vi "Set_DoublePulse_Delay.vi"(8 "error in":errorcluster, 9 "WaitForReady":bool, 10 "InputParams.":variant) -> (0 "error out":errorcluster, 2 "DP_StagePos.":variant)   [LabVIEW 2013]
uses:
  <instrlib>/ESP300/Public/Data/ESP300_State.ctl
  <instrlib>/ESP300/ESP300.lvlib
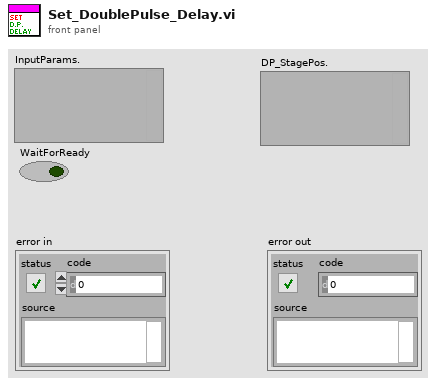
[diagram p1: front panel]
types:
  T1 = cluster{"MotionStageRefs":refnum<queue>, "Axis#":i32, "Delay(ps)":dbl, "ZeroDelay_Offset":dbl}
  T2 = typedef "ESP300.lvlib/ESP300_State.ctl" = cluster{"State":enum16{"Initialize", "SetDefaultConfig", "Close", "Quit", "Identify", "MoveAbs", "MoveAbs_all", "MoveRel", "MoveRel_all", "STOP", "Origin/Home", "WaitStop", "QueryStatus", "UpdateXPos", "UpdateAll", "SetVelocity", "SetAcceleration", "ClearErr", "LogMessage", "MotorEnable(1)", "EnableAxis", "JoyStick", "GetVelocity", "GetAcceleration", "SendCmd", "SetSoftLimits", "Beep", "_SettingReturn", "SoftReset"}, "Params.":variant}
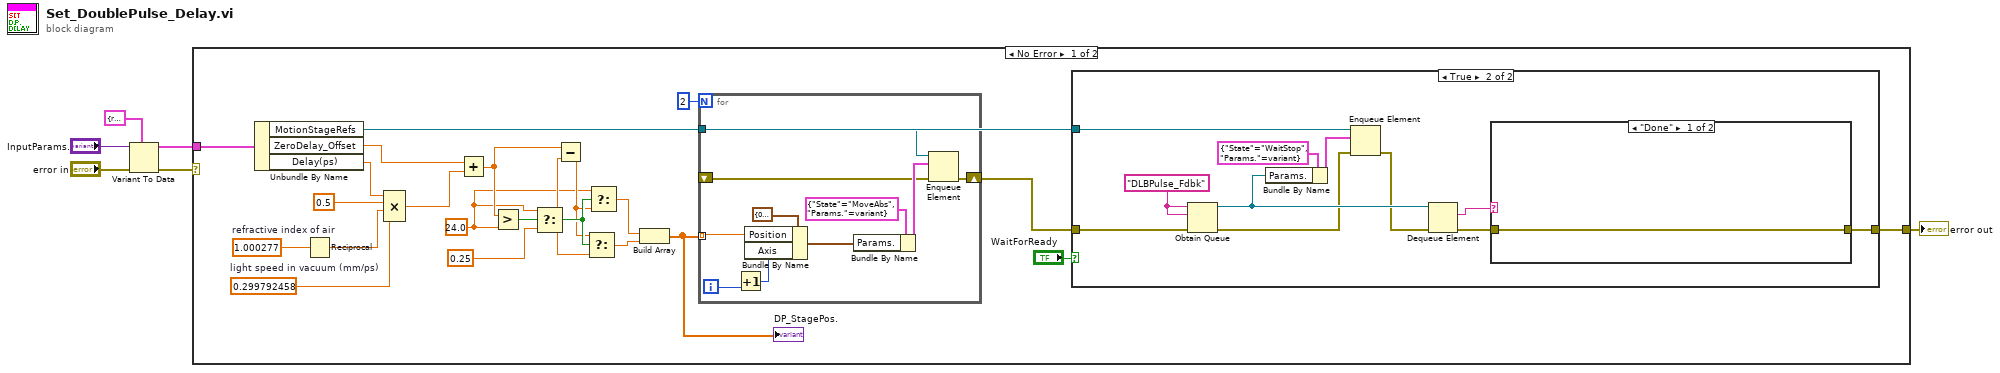
[diagram p0: block diagram]
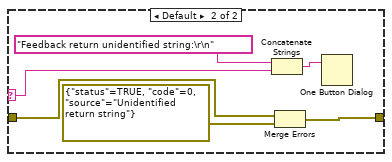
[diagram p3: hidden frame]
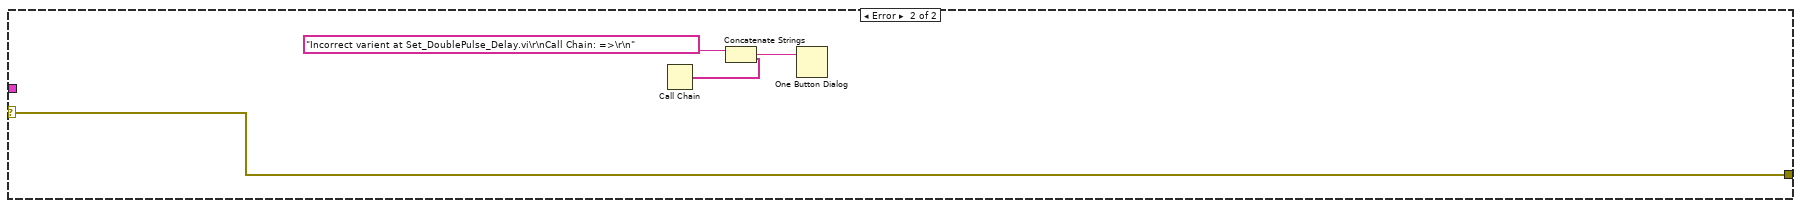
[diagram p4: hidden frame]
diagram:
  n1 = Variant To Data(error in="error in", type=T1 {"MotionStageRefs"=refnum, "Axis#"=0, "Delay(ps)"=0.0, "ZeroDelay_Offset"=0.0} ("Params."), Variant="InputParams.") -> (data=w4:T1, error out=w3:errorcluster)
  n2 = case shown="No Error" w3 {
    selector: w3 -> [_ w58]
    tunnel: w4 -> [w24 _]
    tunnel: [w21 w58] -> w2
    frame No Error {
      w9 = 24.0 ("y")
      w27 = 0.299792458  # light speed in vacuum (mm/ps)
      w7 = 1.000277  # refractive index of air
      n3 = Unbundle By Name(w24) -> ("MotionStageRefs"=w23:refnum<queue>, "ZeroDelay_Offset"=w10:dbl, "Delay(ps)"=w25:dbl)
      n4 = Reciprocal(x=w7) -> (1/x=w26:dbl)
      n5 = Compound Arithmetic op=MULTIPLY(w25, 0.5, w26, w27) -> (w11:dbl)
      n6 = Add(x=w10, y=w11) -> (x+y=w18:dbl)
      n7 = Greater?(x=w18, y=w9) -> (0:w16:bool)
      n8 = Select(t=w9, s=w16, f=0.25) -> (s? t:f=w12:dbl)
      n9 = Subtract(x=w18, y=w12) -> (x-y=w13:dbl)
      n10 = Select(t=w13, s=w16, f=w12) -> (s? t:f=w14:dbl)
      n11 = Select(t=w9, s=w16, f=w13) -> (s? t:f=w15:dbl)
      n12 = Build Array(w15, w14) -> (w8:dbl[])
      "DP_StagePos." <- w8
      n13 = for {
        N: 2 -> [_]
        tunnel: w23 -> [w34]
        shift-right: [w33] -> w20
        shift-left: _ -> [w32]
        tunnel: w8 -> [w30] mode=indexing
        i -> [w31]
        n14 = Increment(x=w31) -> (x+1=w29:i32)
        n15 = Bundle By Name(cluster=cluster{"Axis":i32, "Position":dbl} {"Axis"=0, "Position"=0.0}, "Position"=w30, "Axis"=w29) -> (w35:cluster{"Axis":i32, "Position":dbl})
        n16 = Bundle By Name(cluster=T2 {"State"=enum."MoveAbs", "Params."=variant} ("element"), "Params."=w35) -> (w37:T2)
        n17 = Enqueue Element(queue=w34, element=w37, error in (no error)=w32) -> (error out=w33:errorcluster)  [unwired: 1 in, 2 out]
      }
      n18 = case shown="True" "WaitForReady" {
        tunnel: w23 -> [_ w50]
        tunnel: [w39 w41] -> w21
        tunnel: w20 -> [w39 w40]
        frame False {
        }
        frame True {
          w44 = "DLBPulse_Fdbk" ("name (unnamed)")
          n19 = Obtain Queue(name (unnamed)=w44, element data type=w44, error in (no error)=w40) -> (queue out=w47:refnum<queue>, error out=w45:errorcluster)  [unwired: 2 in, 1 out]
          n20 = Bundle By Name(cluster=T2 {"State"=enum."WaitStop", "Params."=variant} ("element"), "Params."=w47) -> (w48:T2)
          n21 = Enqueue Element(queue=w50, element=w48, error in (no error)=w45) -> (error out=w46:errorcluster)  [unwired: 1 in, 2 out]
          n22 = Dequeue Element(queue=w47, error in (no error)=w46) -> (element=w43:string, error out=w42:errorcluster)  [unwired: 1 in, 2 out]
          n23 = case shown="\"Done\"" w43 {
            selector: w43 -> [_ w55]
            tunnel: w42 -> [w51 w54]
            tunnel: [w51 w52] -> w41
            frame "Done" {
            }
            frame Default {
              n24 = Concatenate Strings("Feedback return unidentified string:\r\n" ("message"), w55) -> (w56:string)
              n25 = Merge Errors(w54, errorcluster {"status"=TRUE, "code"=0, "source"="Unidentified return string"} ("error in")) -> (w52:errorcluster)
              n26 = One Button Dialog(message=w56) -> ()  [unwired: 1 in, 1 out]
            }
          }
        }
      }
    }
    frame Error {
      n27 = Call Chain() -> (call chain=w59:string[])
      n28 = Concatenate Strings("Incorrect varient at Set_DoublePulse_Delay.vi\r\nCall Chain: =>\r\n" ("message"), w59) -> (w60:string)
      n29 = One Button Dialog(message=w60) -> ()  [unwired: 1 in, 1 out]
    }
  }
  "error out" <- w2
